vi "DAQmx Write (Digital U8 1Chan 1Samp).vi"(0 "task/channels in":refnum<k21>, 1 "auto start":bool=TRUE, 7 "data":u8, 9 "timeout":dbl=10.0 format="%0.2f", 11 "error in":errorcluster) -> (4 "task out":refnum<k21>, 10 "number of samples written per channel":u32, 15 "error out":errorcluster)   [LabVIEW 2017]
doc: "Writes a single 8-bit unsigned integer sample to a task that contains a single digital output channel. Use an instance that writes 8-bit unsigned integers for devices with up to eight lines per port."
uses:
  nilvaiu.dll
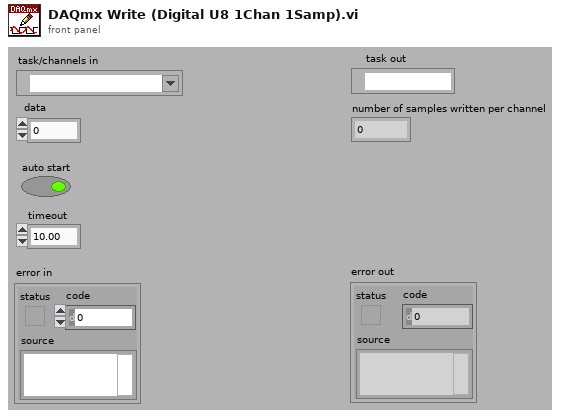
[diagram p1: front panel]
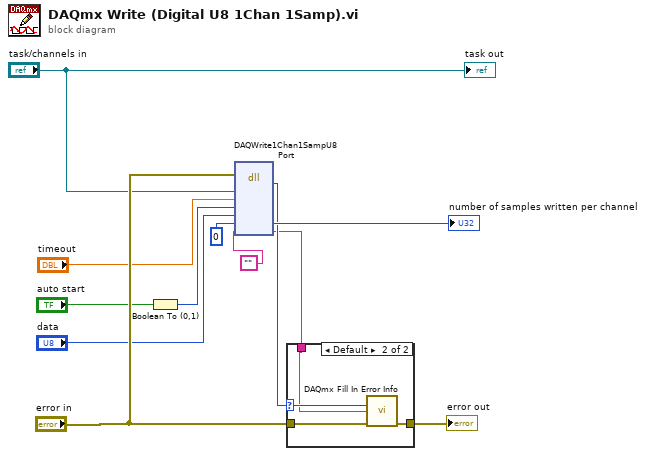
[diagram p0: block diagram]
diagram:
  n1 = Boolean To (0,1)(Boolean="auto start") -> (0, 1=w4:i16)
  n2 = dll-call lib="nilvaiu.*" fn="DAQWrite1Chan1SampU8Port"(error in="error in", "taskID"="task/channels in", "timeout"="timeout", "autoStart"=w4, "data"="data", "numSamplesWriten"=u32 0, "extendedErrorInfo"="") -> (w5:i32, "numSamplesWriten"=→"number of samples written per channel":u32, "extendedErrorInfo"=w3:string)  [unwired: 4 in, 4 out]
  n3 = case shown="Default" w5 {
    selector: w5 -> [_ w15]
    tunnel: "error in" -> [w13 w17]
    tunnel: [w13 w16] -> w10
    tunnel: w3 -> [_ w14]
    frame 0 {
    }
    frame Default {
      n4 = call "DAQmx Fill In Error Info.vi"("status code"=w15, "extended error info"=w14, "error in"=w17) -> ("error out"=w16:errorcluster)  [unwired: 1 in, 11 out]
    }
  }
  "error out" <- w10
  "task out" <- "task/channels in"
